vi "Hello World.vi"(10 "String":string) -> (2 "Msg Strategy":refnum<class "Msg Strategy.lvclass">)   [LabVIEW 2021, in "Hello World Event.lvlib" / "Hello World Msg Strategy.lvlib"]
uses:
  Hello World Msg Strategy.lvlib
  <vilib>/Nathan Davis/jettl/jettl/Msg Strategy/Msg Strategy.lvclass
  Hello World Msg Strategy/Hello World Msg Strategy.lvclass
  C:/Program Files/National Instruments/LabVIEW 2021/vi.lib/Nathan Davis/jettl/jettl/Msg Strategy/Msg Strategy.lvclass
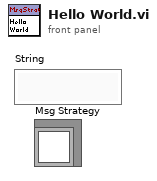
[diagram p1: front panel]
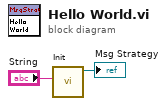
[diagram p0: block diagram]
diagram:
  n1 = call "Init.vi"("String"="String") -> ("Hello World Msg Strategy out"=→"Msg Strategy":refnum<class "Hello World Msg Strategy.lvclass">)  [unwired: 10 in]
